vi "Return Tool.vi"(8 "error in":errorcluster, 11 "Gantry in":refnum<class "Gantry Class.lvclass">) -> (0 "error out":errorcluster, 3 "Gantry out":refnum<class "Gantry Class.lvclass">)   [LabVIEW 2017, in "Gantry Class.lvclass"]
uses:
  Gantry Class.lvclass
  FlexWorktable/FlexWorktable.lvclass
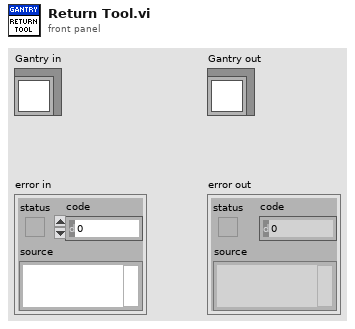
[diagram p1: front panel]
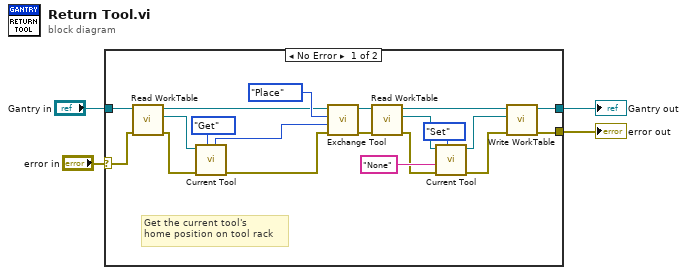
[diagram p0: block diagram]
diagram:
  n1 = case shown="No Error" "error in" {
    selector: "error in" -> [w23 w26]
    tunnel: [w14 w26] -> w1
    tunnel: [w15 w25] -> w2
    tunnel: "Gantry in" -> [w24 w25]
    frame No Error {
      # "Get the current tool's \nhome position on tool rack"
      n2 = call-dynamic "Read WorkTable.vi"("error in"=w23, "Gantry Class in"=w24) -> ("error out"=w19:errorcluster, "Worktable"=w21:refnum<class "FlexWorktable.lvclass">, "Gantry Class out"=w11:refnum<class "Gantry Class.lvclass">)  [unwired: 7 in]
      n3 = call-dynamic "Current Tool.vi"("Get/Set"=enum16{"Get", "Set"}."Get", "error in (no error)"=w19, "FlexWorktable in"=w21) -> ("error out"=w10:errorcluster, "Rack Position"=w18:i32)  [unwired: 5 in, 2 out]
      n4 = call-dynamic "Exchange Tool.vi"("error in"=w10, "Tool Position"=w18, "Place/Pick"=enum16{"Place", "Pick"}."Place", "Gantry in"=w11) -> ("error out"=w9:errorcluster, "Gantry out"=w8:refnum<class "Gantry Class.lvclass">)  [unwired: 6 in]
      n5 = call-dynamic "Read WorkTable.vi"("error in"=w9, "Gantry Class in"=w8) -> ("error out"=w7:errorcluster, "Worktable"=w5:refnum<class "FlexWorktable.lvclass">, "Gantry Class out"=w6:refnum<class "Gantry Class.lvclass">)  [unwired: 7 in]
      n6 = call-dynamic "Current Tool.vi"("Get/Set"=enum16{"Get", "Set"}."Set", "error in (no error)"=w7, "Tool in"="None", "FlexWorktable in"=w5) -> ("error out"=w13:errorcluster, "FlexWorktable out"=w12:refnum<class "FlexWorktable.lvclass">)  [unwired: 4 in, 2 out]
      n7 = call-dynamic "Write WorkTable.vi"("error in (no error)"=w13, "FlexWorktable"=w12, "Gantry Class in"=w6) -> ("error out"=w14:errorcluster, "Gantry Class out"=w15:refnum<class "Gantry Class.lvclass">)  [unwired: 7 in]
    }
    frame Error {
    }
  }
  "error out" <- w1
  "Gantry out" <- w2
